vi "detector_acquire_generic_data.vi"(8 "error in (no error)":errorcluster, 11 "detector in":refnum<class "detector.lvclass">) -> (0 "error out":errorcluster, 2 "image_data":T1, 3 "detector out":refnum<class "detector.lvclass">)   [LabVIEW 2015, in "detector.lvclass"]
uses:
  detector.lvclass
  Experiment/experiment_panel/2d_scan/detector_data_tdef.ctl
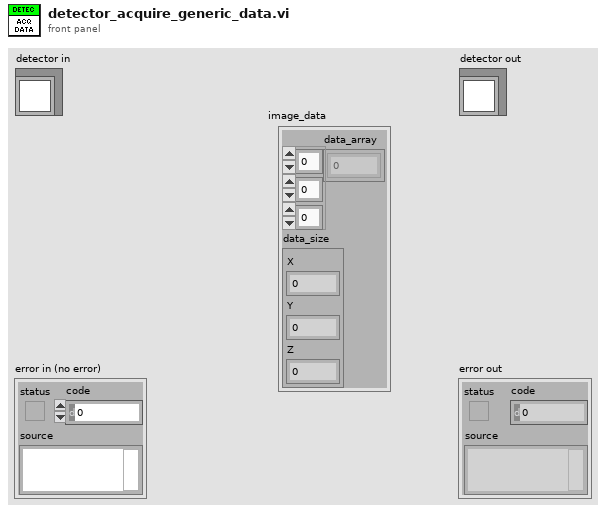
[diagram p1: front panel]
types:
  T1 = typedef "detector_data_tdef.ctl" = cluster{"data_array":dbl[][][], "data_size":cluster{"X":i32, "Y":i32, "Z":i32}}
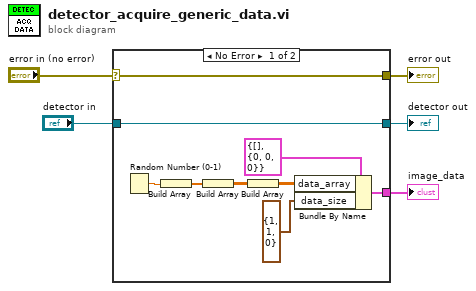
[diagram p0: block diagram]
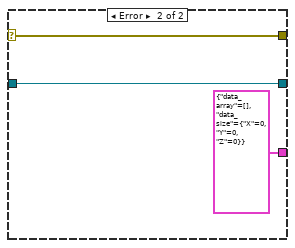
[diagram p2: hidden frame]
diagram:
  n1 = case shown="No Error" "error in (no error)" {
    selector: "error in (no error)" -> [w13 w17]
    tunnel: [w13 w17] -> w4
    tunnel: [w14 w16] -> w2
    tunnel: "detector in" -> [w14 w16]
    tunnel: [w6 T1 {"data_array"=[], "data_size"={"X"=0, "Y"=0, "Z"=0}} ("image_data")] -> w1
    frame No Error {
      n2 = Random Number (0-1)() -> (number: 0 to 1=w11:dbl)
      n3 = Build Array(w11) -> (w10:dbl[])
      n4 = Build Array(w10) -> (w9:dbl[][])
      n5 = Build Array(w9) -> (w8:dbl[][][])
      n6 = Bundle By Name(cluster=T1 {"data_array"=[], "data_size"={"X"=0, "Y"=0, "Z"=0}} ("image_data"), "data_array"=w8, "data_size"=cluster{"X":i32, "Y":i32, "Z":i32} {"X"=1, "Y"=1, "Z"=0}) -> (w6:T1)
    }
    frame Error {
    }
  }
  "error out" <- w4
  "detector out" <- w2
  "image_data" <- w1
